vi "Spaceship_Move.vi"(1 "Spaceship_data in":T1) -> (0 "Spaceship_data out":T1)   [LabVIEW 2017]
uses:
  Spaceship_data.ctl
  GameConfig/GameConfig_data.ctl
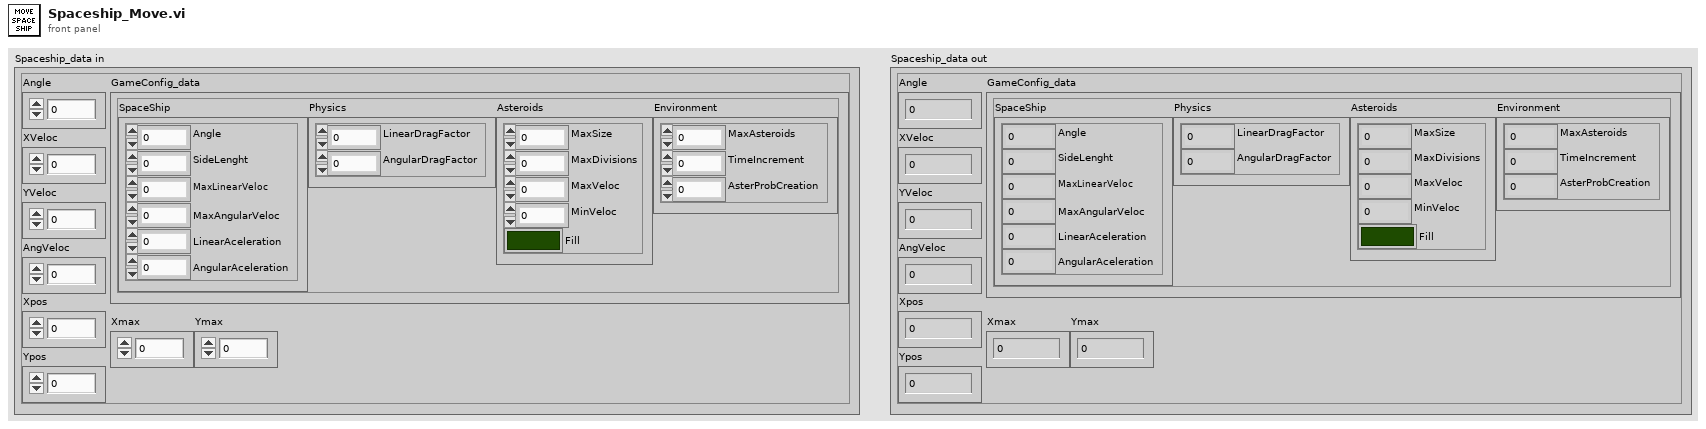
[diagram p1: front panel]
types:
  T1 = typedef "Spaceship_data.ctl" = cluster{"Angle":dbl, "XVeloc":dbl, "YVeloc":dbl, "AngVeloc":dbl, "GameConfig_data":T2, "Xpos":dbl, "Ypos":dbl, "Xmax":dbl, "Ymax":dbl}
  T2 = typedef "GameConfig_data.ctl" = cluster{"SpaceShip":cluster{"Angle":dbl, "SideLenght":dbl, "MaxLinearVeloc":dbl, "MaxAngularVeloc":dbl, "LinearAceleration":dbl, "AngularAceleration":dbl}, "Physics":cluster{"LinearDragFactor":dbl, "AngularDragFactor":dbl}, "Asteroids":cluster{"MaxSize":dbl, "MaxDivisions":i32, "MaxVeloc":dbl, "MinVeloc":dbl, "Fill":bool}, "Environment":cluster{"MaxAsteroids":i32, "TimeIncrement":dbl, "AsterProbCreation":dbl}}
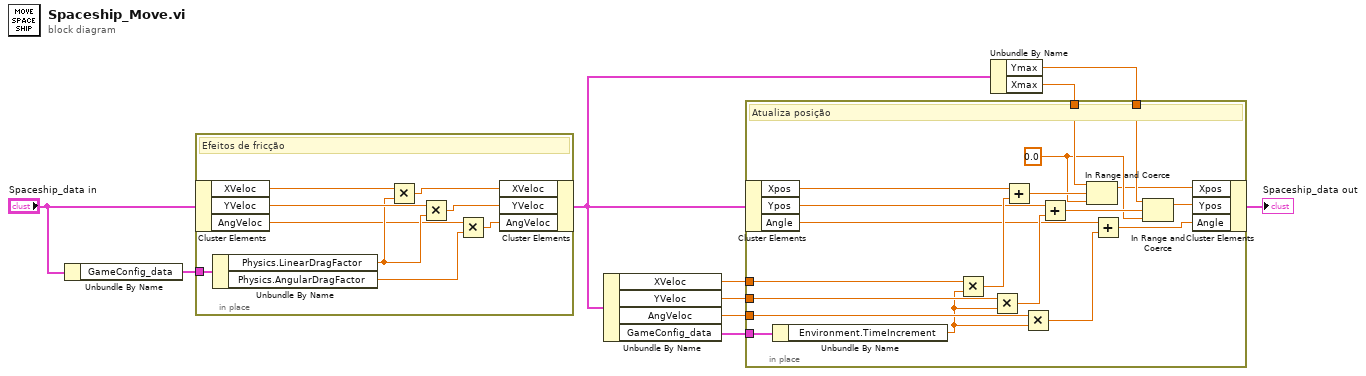
[diagram p0: block diagram]
diagram:
  n1 = Unbundle By Name("Spaceship_data in") -> ("GameConfig_data"=w5:T2)
  n2 = in-place {
    in-place-border: w5 -> [w19]
    # "Efeitos de fricção"
    n3 = in-place-cluster #1("Spaceship_data in") -> ("XVeloc"=w18:dbl, "YVeloc"=w16:dbl, "AngVeloc"=w13:dbl)
    n4 = Unbundle By Name(w19) -> ("Physics.LinearDragFactor"=w15:dbl, "Physics.AngularDragFactor"=w11:dbl)
    n5 = Multiply(x=w18, y=w15) -> (x*y=w17:dbl)
    n6 = Multiply(x=w16, y=w15) -> (x*y=w14:dbl)
    n7 = Multiply(x=w13, y=w11) -> (x*y=w12:dbl)
    n8 = in-place-cluster #1("XVeloc"=w17, "YVeloc"=w14, "AngVeloc"=w12) -> (w3:T1)
  }
  n9 = Unbundle By Name(w3) -> ("XVeloc"=w7:dbl, "YVeloc"=w8:dbl, "AngVeloc"=w9:dbl, "GameConfig_data"=w6:T2)
  n10 = Unbundle By Name(w3) -> ("Ymax"=w1:dbl, "Xmax"=w2:dbl)
  n11 = in-place {
    in-place-border: w6 -> [w38]
    in-place-border: w7 -> [w37]
    in-place-border: w8 -> [w34]
    in-place-border: w9 -> [w31]
    in-place-border: w2 -> [w25]
    in-place-border: w1 -> [w22]
    w21 = 0.0 ("lower limit")
    # "Atualiza posição"
    n12 = in-place-cluster #2(w3) -> ("Xpos"=w36:dbl, "Ypos"=w33:dbl, "Angle"=w29:dbl)
    n13 = Unbundle By Name(w38) -> ("Environment.TimeIncrement"=w30:dbl)
    n14 = Multiply(x=w37, y=w30) -> (x*y=w35:dbl)
    n15 = Multiply(x=w34, y=w30) -> (x*y=w32:dbl)
    n16 = Add(x=w36, y=w35) -> (x+y=w26:dbl)
    n17 = Multiply(x=w31, y=w30) -> (x*y=w28:dbl)
    n18 = Add(x=w33, y=w32) -> (x+y=w24:dbl)
    n19 = In Range and Coerce(upper limit=w25, x=w26, lower limit=w21) -> (coerced(x)=w20:dbl)  [unwired: 1 out]
    n20 = Add(x=w29, y=w28) -> (x+y=w27:dbl)
    n21 = In Range and Coerce(upper limit=w22, x=w24, lower limit=w21) -> (coerced(x)=w23:dbl)  [unwired: 1 out]
    n22 = in-place-cluster #2("Xpos"=w20, "Ypos"=w23, "Angle"=w27) -> (→"Spaceship_data out":T1)
  }
